vi "Read Rank.vi"(8 "error in (no error)":errorcluster, 11 "SA 54GHz Path Group in":refnum<class "SA 54GHz Path Group.lvclass">) -> (0 "error out":errorcluster, 2 "Rank":dbl, 3 "SA 54GHz Path Group out":refnum<class "SA 54GHz Path Group.lvclass">)   [LabVIEW 2023, in "RFFixtureCharact.RMM.lvlib" / "SA 54GHz Path Group.lvclass"]
uses:
  SA 54GHz Path Group.lvclass
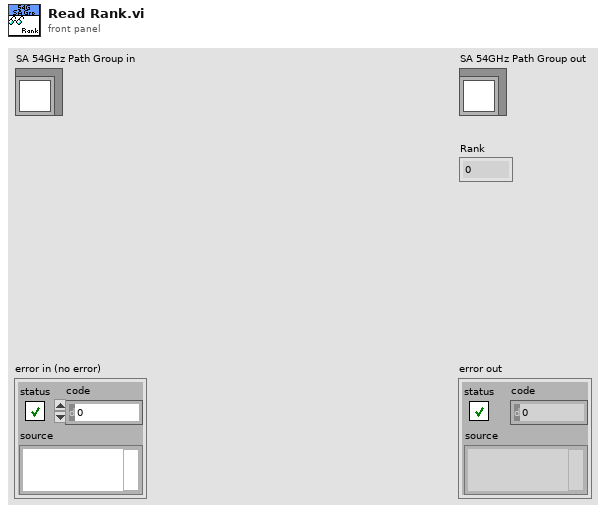
[diagram p1: front panel]
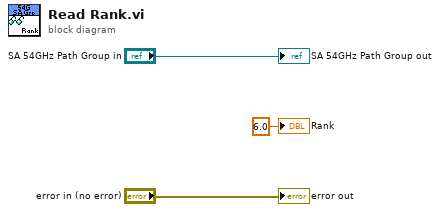
[diagram p0: block diagram]
diagram:
  "error out" <- "error in (no error)"
  "SA 54GHz Path Group out" <- "SA 54GHz Path Group in"
  "Rank" <- 6.0 ("Rank")
